vi "Error - Log Error.vi"(8 "error in (no error)":errorcluster, 10 "Variant":variant, 11 "Error Type":T1) -> (0 "error out":errorcluster)   [LabVIEW 2017]
doc: "This SubVI store error information to external Log file"
uses:
  Controls/Error Type.ctl
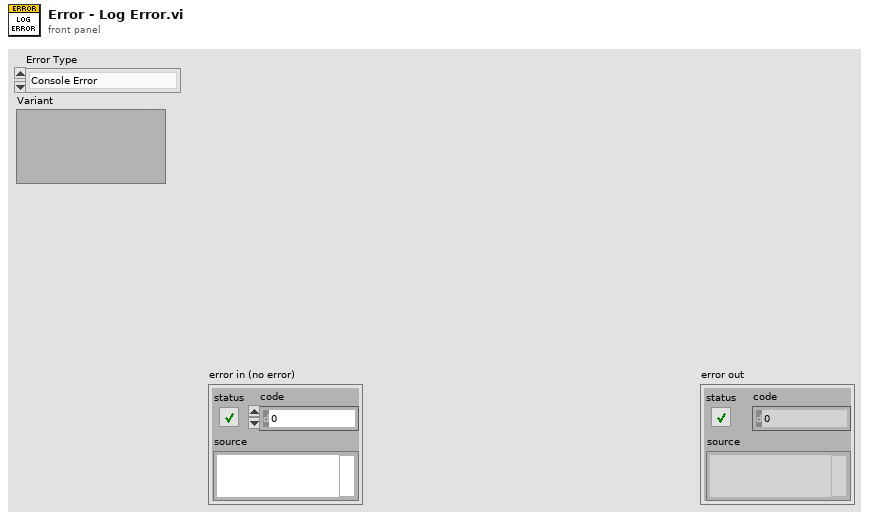
[diagram p1: front panel]
types:
  T1 = typedef "Error Type.ctl" = enum16{"Console Error", "Process Step Error", "Sensor Interface IO Error"}
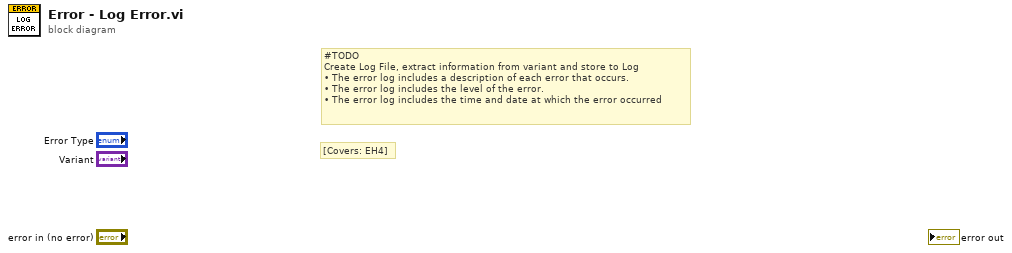
[diagram p0: block diagram]
diagram:
  # "[Covers: EH4]"
  # "#TODO\nCreate Log File, extract information from variant and store to Log\n• The error log includes a description of each error that occurs.\n• The error log includes the level of the error.\n• The error log includes the time and date at which the error occurred"
